vi "Update Data Plot.vi"(6 "Sample Rate (sec/sample)":dbl, 8 "Time interval (s)":i32, 9 "Instrument State":T2 {"Instrument State"."Temperature (C)" min=0}, 10 "History length (-1; unlimited)":i32=-1, 11 "Graph History Arrays in":T1) -> (0 "Updated Plot History":cluster{timestamp[], dbl[]}[](array[cluster]), 3 "Graph History Arrays out":T1)   [LabVIEW 2020, in "plugin_flodx_ph_probe.lvlib" / "plugin.lvlib"]
uses:
  plugin.lvlib
  Instrument Manager/loop/Instrument Loop State.ctl
  Instrument Manager/connection_info/Connection Info.ctl
  Instrument Manager/Instrument State.ctl
  Data Display Loop Data.ctl
  Instrument Manager/Instrument Manager.lvlib
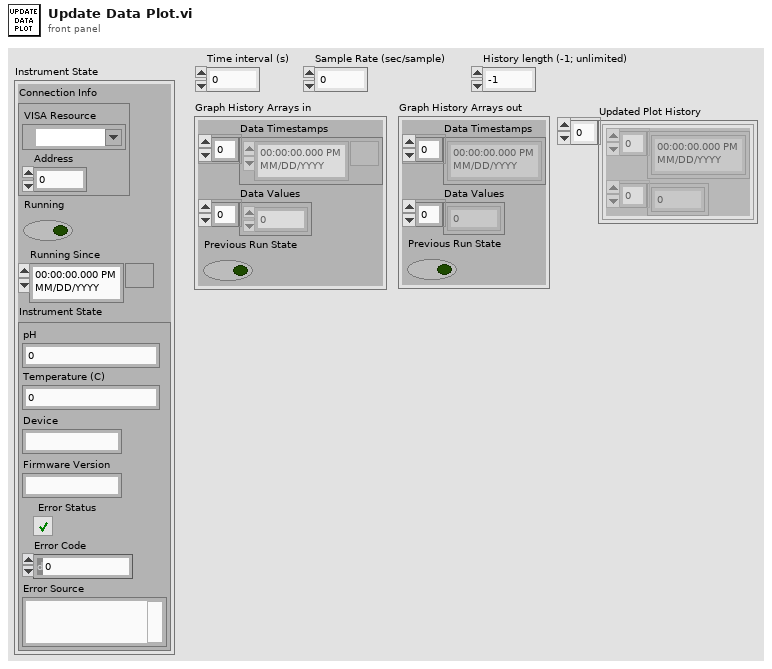
[diagram p1: front panel]
types:
  T1 = typedef "plugin_flodx_ph_probe.lvlib/plugin.lvlib/Data Display Loop Data.ctl" = cluster{"Data Timestamps":timestamp[], "Data Values":dbl[], "Previous Run State":bool}
  T2 = typedef "plugin_flodx_ph_probe.lvlib/plugin.lvlib/Instrument Manager.lvlib/Instrument Loop State.ctl" = cluster{"Connection Info":T3, "Running":bool, "Running Since":timestamp, "Instrument State":T4}
  T3 = typedef "plugin_flodx_ph_probe.lvlib/plugin.lvlib/Instrument Manager.lvlib/Connection Info.ctl" = cluster{"VISA Resource":refnum<visa-resource-name>, "Address":u8}
  T4 = typedef "plugin_flodx_ph_probe.lvlib/plugin.lvlib/Instrument Manager.lvlib/Instrument State.ctl" = cluster{"pH":sgl, "Temperature (C)":sgl, "Device":string, "Firmware Version":string, "Error Status":bool, "Error Code":i32, "Error Source":string}
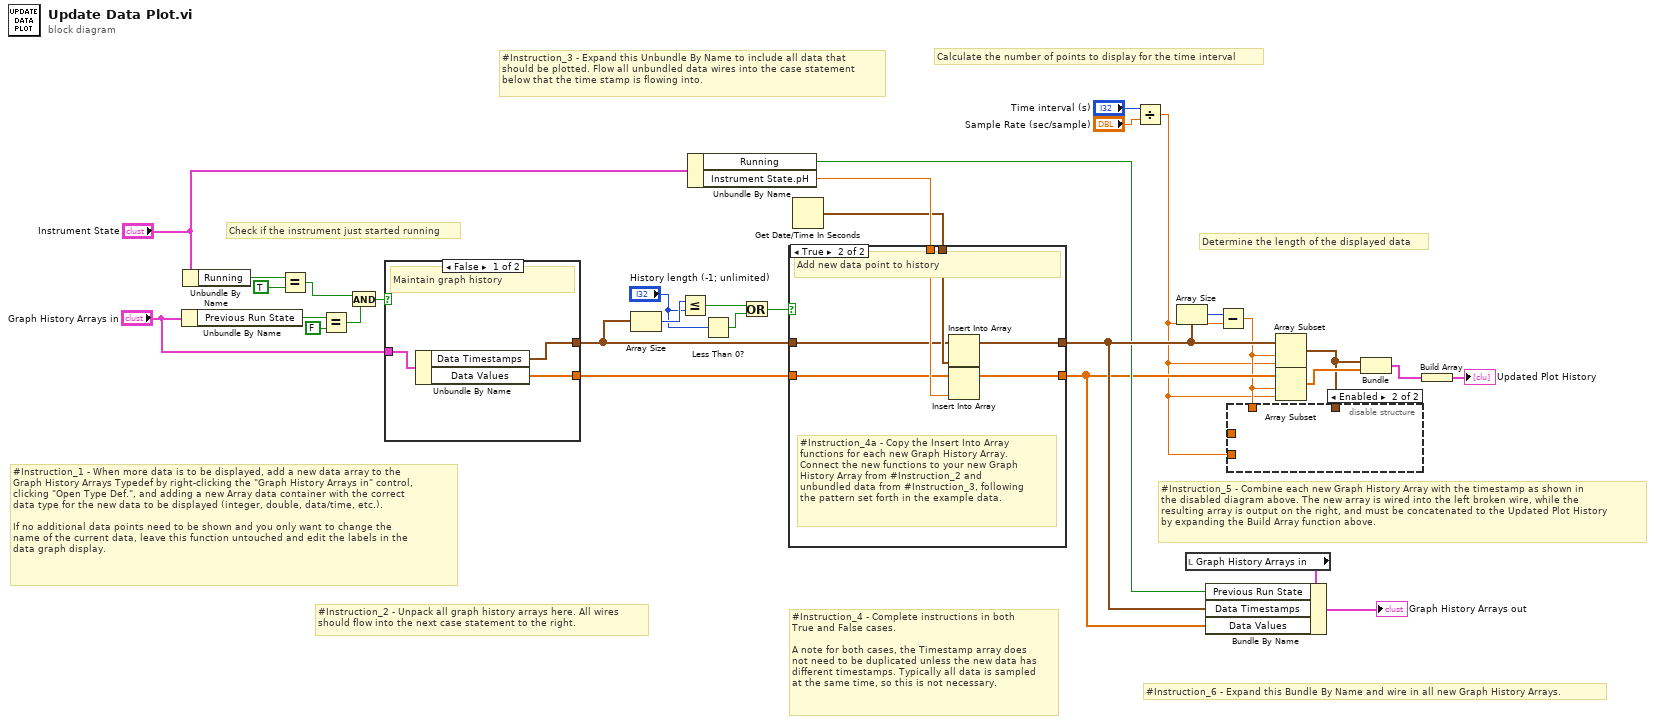
[diagram p0: block diagram]
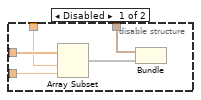
[diagram p2: hidden frame]
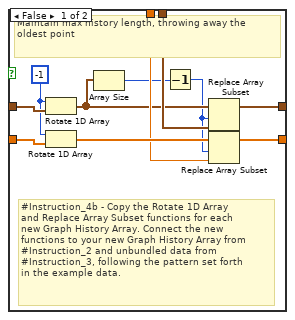
[diagram p3: hidden frame]
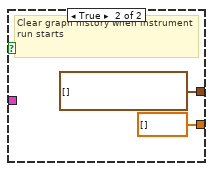
[diagram p4: hidden frame]
diagram:
  # "#Instruction_6 - Expand this Bundle By Name and wire in all new Graph History Arrays."
  # "#Instruction_5 - Combine each new Graph History Array with the timestamp as shown in\nthe disabled diagram above. The new array is wired into the left broken wire, while the \nresulting array is output on the right, and must be concatenated to the Updated Plot History\nby expanding the Build Array function above."
  # "#Instruction_4 - Complete instructions in both\nTrue and False cases.\n\nA note for both cases, the Timestamp array does \nnot need to be duplicated unless the new data has\ndifferent timestamps. Typically all data is sampled \nat the same time, so this is not necessary."
  # "#Instruction_2 - Unpack all graph history arrays here. All wires\nshould flow into the next case statement to the right."
  # "#Instruction_1 - When more data is to be displayed, add a new data array to the\nGraph History Arrays Typedef by right-clicking the \"Graph History Arrays in\" control,\nclicking \"Open Type Def.\", and adding a new Array data container with the correct\ndata type for the new data to be displayed (integer, double, data/time, etc.).\n\nIf no additional data points need to be shown and you only want to change the \nname of the current data, leave this function untouched and edit the labels in the\ndata graph display."
  # "#Instruction_3 - Expand this Unbundle By Name to include all data that\nshould be plotted. Flow all unbundled data wires into the case statement\nbelow that the time stamp is flowing into."
  # "Check if the instrument just started running"
  # "Calculate the number of points to display for the time interval"
  # "Determine the length of the displayed data"
  n1 = Unbundle By Name("Graph History Arrays in") -> ("Previous Run State"=w21:bool)
  n2 = Unbundle By Name("Instrument State") -> ("Running"=w27:bool)
  n3 = Equal?(x=w27, y=TRUE) -> (x = y?=w17:bool)
  n4 = Equal?(x=w21, y=FALSE) -> (x = y?=w18:bool)
  n5 = And(x=w17, y=w18) -> (x .and. y?=w19:bool)
  n6 = case shown="False" w19 {
    tunnel: "Graph History Arrays in" -> [w35 _]
    tunnel: [w34 dbl[] [] ("Data Values")] -> w23
    tunnel: [w33 timestamp[] [] ("Data Timestamps")] -> w13
    frame False {
      # "Maintain graph history"
      n7 = Unbundle By Name(w35) -> ("Data Timestamps"=w33:timestamp[], "Data Values"=w34:dbl[])
    }
    frame True {
      # "Clear graph history when instrument run starts"
    }
  }
  n8 = Array Size(array=w13) -> (size(s)=w12:i32)
  n9 = Less Or Equal?(x=w12, y="History length (-1; unlimited)") -> (x <= y?=w9:bool)
  n10 = Unbundle By Name("Instrument State") -> ("Running"=w14:bool, "Instrument State.pH"=w24:sgl)
  n11 = Less Than 0?(x="History length (-1; unlimited)") -> (x < 0?=w10:bool)
  n12 = Or(x=w9, y=w10) -> (x .or. y?=w8:bool)
  n13 = Get Date/Time In Seconds() -> (seconds since 1Jan1904=w1:timestamp)
  n14 = case shown="True" w8 {
    tunnel: [w39 w54] -> w26
    tunnel: [w38 w53] -> w5
    tunnel: w1 -> [w43 w52]
    tunnel: w24 -> [w44 w51]
    tunnel: w23 -> [w47 w50]
    tunnel: w13 -> [w48 w49]
    frame False {
      w46 = -1
      # "#Instruction_4b - Copy the Rotate 1D Array \nand Replace Array Subset functions for each\nnew Graph History Array. Connect the new\nfunctions to your new Graph History Array from\n#Instruction_2 and unbundled data from\n#Instruction_3, following the pattern set forth\nin the example data."
      # "Maintain max history length, throwing away the oldest point"
      n15 = Rotate 1D Array(1:w48, 2:w46) -> (0:w42:timestamp[])
      n16 = Rotate 1D Array(1:w47, 2:w46) -> (0:w45:dbl[])
      n17 = Array Size(array=w42) -> (size(s)=w41:i32)
      n18 = Decrement(x=w41) -> (x-1=w40:i32)
      n19 = Replace Array Subset(array=w42, new element=w43, index=w40) -> (w39:timestamp[])
      n20 = Replace Array Subset(array=w45, new element=w44, index=w40) -> (w38:dbl[])
    }
    frame True {
      # "#Instruction_4a - Copy the Insert Into Array \nfunctions for each new Graph History Array. \nConnect the new functions to your new Graph \nHistory Array from #Instruction_2 and \nunbundled data from #Instruction_3, following \nthe pattern set forth in the example data."
      # "Add new data point to history"
      n21 = Insert Into Array(array=w49, new element=w52) -> (w54:timestamp[])  [unwired: 1 in]
      n22 = Insert Into Array(array=w50, new element=w51) -> (w53:dbl[])  [unwired: 1 in]
    }
  }
  n23 = Divide(x="Time interval (s)", y="Sample Rate (sec/sample)") -> (x/y=w2:dbl)
  n24 = Array Size(array=w26) -> (size(s)=w31:i32)
  n25 = local read "Graph History Arrays in"() -> (w25:T1)
  n26 = Bundle By Name(cluster=w25, "Previous Run State"=w14, "Data Timestamps"=w26, "Data Values"=w5) -> (→"Graph History Arrays out":T1)
  n27 = Subtract(x=w31, y=w2) -> (x-y=w3:dbl)
  n28 = Array Subset(array=w26, index=w3, length=w2) -> (w4:timestamp[])
  n29 = disable-structure shown="Enabled" {
    disable-tunnel: _ -> [w59 _]
    disable-tunnel: w4 -> [w57 _]
    disable-tunnel: w3 -> [w56 _]
    disable-tunnel: w2 -> [w55 _]
    frame Disabled {
      n30 = Array Subset(array=w59, index=w56, length=w55) -> (w58:void[])
      n31 = Bundle(w57, w58) -> ()  [unwired: 1 in, 1 out]
    }
    frame Enabled {
    }
  }
  n32 = Array Subset(array=w5, index=w3, length=w2) -> (w30:dbl[])
  n33 = Bundle(w4, w30) -> (w16:cluster{timestamp[], dbl[]})  [unwired: 1 in]
  n34 = Build Array(w16) -> (→"Updated Plot History":cluster{timestamp[], dbl[]}[])
